vi "ps180-Rnn.vi"(3 "error in (no error)":errorcluster, 4 "Polarity":bool, 5 "Read parameter":u16 max=21 step=1, 6 "VISA session":refnum<visa-resource-name>) -> (0 "error out":errorcluster, 1 "Output string":string)   [LabVIEW 2019]
panel:
  # "Rnn, not exactly"
  # "This Vi is a kludge, don't use this to read any parameters.\nI wrote this to clone a particular operation. The numbers \nunder \"Read parameter\" don't correspond to the Rnn command\nnumbers. - MVC"
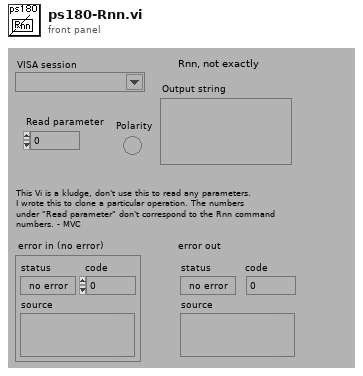
[diagram p1: front panel]
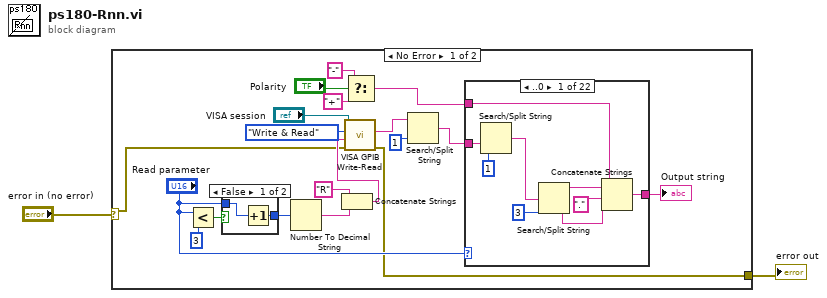
[diagram p0: block diagram]
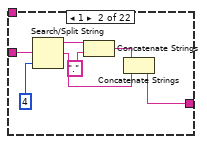
[diagram p3: hidden frame]
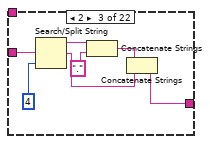
[diagram p4: hidden frame]
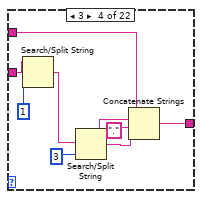
[diagram p5: hidden frame]
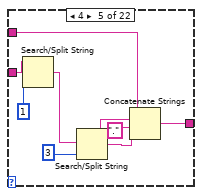
[diagram p6: hidden frame]
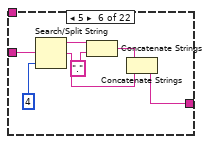
[diagram p7: hidden frame]
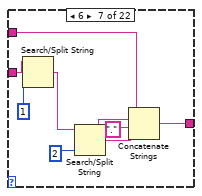
[diagram p8: hidden frame]
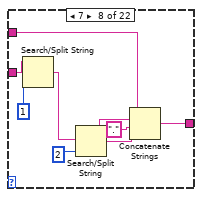
[diagram p9: hidden frame]
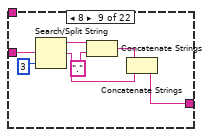
[diagram p10: hidden frame]
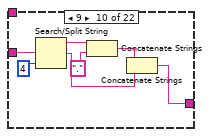
[diagram p11: hidden frame]
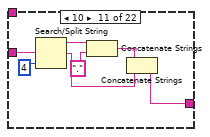
[diagram p12: hidden frame]
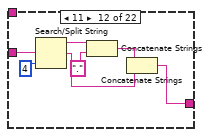
[diagram p13: hidden frame]
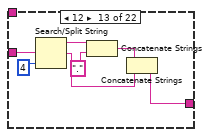
[diagram p14: hidden frame]
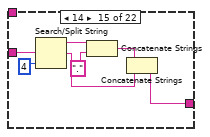
[diagram p16: hidden frame]
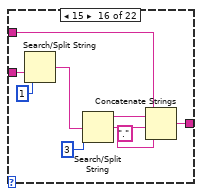
[diagram p17: hidden frame]
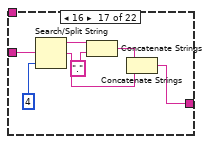
[diagram p18: hidden frame]
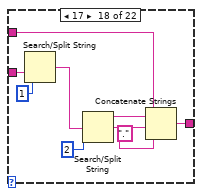
[diagram p19: hidden frame]
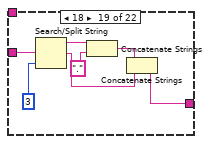
[diagram p20: hidden frame]
diagram:
  n1 = case shown="No Error" "error in (no error)" {
    selector: "error in (no error)" -> [w3 w181]
    tunnel: [w6 w181] -> w2
    frame No Error {
      n2 = Less?(x="Read parameter", y=u16 3) -> (x < y?=w10:bool)
      n3 = case shown="False" w10 {
        tunnel: "Read parameter" -> [w22 w24]
        tunnel: [w23 w24] -> w11
        frame False {
          n4 = Increment(x=w22) -> (x+1=w23:u16)
        }
        frame True {
        }
      }
      n5 = Number To Decimal String(number=w11) -> (decimal integer string=w12:string)  [unwired: 1 in]
      n6 = Concatenate Strings("R", w12) -> (w8:string)
      n7 = call "VISA GPIB Write-Read.vi"("error in (no error)"=w3, "Command"=w8, "Action"=enum16{"Write", "Read", "Write & Read"}."Write & Read", "VISA resource name"="VISA session") -> ("error out"=w6:errorcluster, "String Returned"=w7:string)  [unwired: 4 in, 2 out]
      n8 = Select(t="-", s="Polarity", f="+") -> (s? t:f=w19:string)
      n9 = Search/Split String(string=w7, offset (0)=1) -> (match + rest of string=w16:string)  [unwired: 1 in, 2 out]
      n10 = case shown="..0" "Read parameter" {
        tunnel: w16 -> [w30 w40 w42 w51 w60 w67 w76 w85 w92 w99 w106 w113 w120 w126 w128 w139 w144 w155 w160 w166 w168 w175]
        tunnel: [w28 w34 w41 w53 w62 w66 w78 w87 w91 w98 w105 w112 w119 w126 w127 w137 w143 w153 w159 w166 w167 w174] -> w17
        tunnel: w19 -> [w25 _ _ w48 w57 _ w73 w82 _ _ _ _ _ _ _ w134 _ w150 _ _ _ _]
        frame ..0 {
          n11 = Search/Split String(string=w30, offset (0)=1) -> (match + rest of string=w29:string)  [unwired: 1 in, 2 out]
          n12 = Search/Split String(string=w29, offset (0)=3) -> (substring before match=w27:string, match + rest of string=w26:string)  [unwired: 1 in, 1 out]
          n13 = Concatenate Strings(w25, w27, ".", w26) -> (w28:string)
        }
        frame 1 {
          n14 = Search/Split String(string=w40, offset (0)=4) -> (substring before match=w38:string, match + rest of string=w35:string)  [unwired: 1 in, 1 out]
          n15 = Concatenate Strings(w38, ".") -> (w36:string)
          n16 = Concatenate Strings(w36, w35) -> (w34:string)
        }
        frame 2 {
          n17 = Search/Split String(string=w42, offset (0)=4) -> (substring before match=w46:string, match + rest of string=w43:string)  [unwired: 1 in, 1 out]
          n18 = Concatenate Strings(w46, ".") -> (w44:string)
          n19 = Concatenate Strings(w44, w43) -> (w41:string)
        }
        frame 3 {
          n20 = Search/Split String(string=w51, offset (0)=1) -> (match + rest of string=w50:string)  [unwired: 1 in, 2 out]
          n21 = Search/Split String(string=w50, offset (0)=3) -> (substring before match=w55:string, match + rest of string=w52:string)  [unwired: 1 in, 1 out]
          n22 = Concatenate Strings(w48, w55, ".", w52) -> (w53:string)
        }
        frame 4 {
          n23 = Search/Split String(string=w60, offset (0)=1) -> (match + rest of string=w59:string)  [unwired: 1 in, 2 out]
          n24 = Search/Split String(string=w59, offset (0)=3) -> (substring before match=w64:string, match + rest of string=w61:string)  [unwired: 1 in, 1 out]
          n25 = Concatenate Strings(w57, w64, ".", w61) -> (w62:string)
        }
        frame 5 {
          n26 = Search/Split String(string=w67, offset (0)=4) -> (substring before match=w71:string, match + rest of string=w68:string)  [unwired: 1 in, 1 out]
          n27 = Concatenate Strings(w71, ".") -> (w69:string)
          n28 = Concatenate Strings(w69, w68) -> (w66:string)
        }
        frame 6 {
          n29 = Search/Split String(string=w76, offset (0)=1) -> (match + rest of string=w75:string)  [unwired: 1 in, 2 out]
          n30 = Search/Split String(string=w75, offset (0)=2) -> (substring before match=w80:string, match + rest of string=w77:string)  [unwired: 1 in, 1 out]
          n31 = Concatenate Strings(w73, w80, ".", w77) -> (w78:string)
        }
        frame 7 {
          n32 = Search/Split String(string=w85, offset (0)=1) -> (match + rest of string=w84:string)  [unwired: 1 in, 2 out]
          n33 = Search/Split String(string=w84, offset (0)=2) -> (substring before match=w89:string, match + rest of string=w86:string)  [unwired: 1 in, 1 out]
          n34 = Concatenate Strings(w82, w89, ".", w86) -> (w87:string)
        }
        frame 8 {
          n35 = Search/Split String(string=w92, offset (0)=3) -> (substring before match=w96:string, match + rest of string=w93:string)  [unwired: 1 in, 1 out]
          n36 = Concatenate Strings(w96, ".") -> (w94:string)
          n37 = Concatenate Strings(w94, w93) -> (w91:string)
        }
        frame 9 {
          n38 = Search/Split String(string=w99, offset (0)=4) -> (substring before match=w103:string, match + rest of string=w100:string)  [unwired: 1 in, 1 out]
          n39 = Concatenate Strings(w103, ".") -> (w101:string)
          n40 = Concatenate Strings(w101, w100) -> (w98:string)
        }
        frame 10 {
          n41 = Search/Split String(string=w106, offset (0)=4) -> (substring before match=w110:string, match + rest of string=w107:string)  [unwired: 1 in, 1 out]
          n42 = Concatenate Strings(w110, ".") -> (w108:string)
          n43 = Concatenate Strings(w108, w107) -> (w105:string)
        }
        frame 11 {
          n44 = Search/Split String(string=w113, offset (0)=4) -> (substring before match=w117:string, match + rest of string=w114:string)  [unwired: 1 in, 1 out]
          n45 = Concatenate Strings(w117, ".") -> (w115:string)
          n46 = Concatenate Strings(w115, w114) -> (w112:string)
        }
        frame 12 {
          n47 = Search/Split String(string=w120, offset (0)=4) -> (substring before match=w124:string, match + rest of string=w121:string)  [unwired: 1 in, 1 out]
          n48 = Concatenate Strings(w124, ".") -> (w122:string)
          n49 = Concatenate Strings(w122, w121) -> (w119:string)
        }
        frame 13 {
        }
        frame 14 {
          n50 = Search/Split String(string=w128, offset (0)=4) -> (substring before match=w132:string, match + rest of string=w129:string)  [unwired: 1 in, 1 out]
          n51 = Concatenate Strings(w132, ".") -> (w130:string)
          n52 = Concatenate Strings(w130, w129) -> (w127:string)
        }
        frame 15 {
          n53 = Search/Split String(string=w139, offset (0)=1) -> (match + rest of string=w138:string)  [unwired: 1 in, 2 out]
          n54 = Search/Split String(string=w138, offset (0)=3) -> (substring before match=w136:string, match + rest of string=w135:string)  [unwired: 1 in, 1 out]
          n55 = Concatenate Strings(w134, w136, ".", w135) -> (w137:string)
        }
        frame 16 {
          n56 = Search/Split String(string=w144, offset (0)=4) -> (substring before match=w148:string, match + rest of string=w145:string)  [unwired: 1 in, 1 out]
          n57 = Concatenate Strings(w148, ".") -> (w146:string)
          n58 = Concatenate Strings(w146, w145) -> (w143:string)
        }
        frame 17 {
          n59 = Search/Split String(string=w155, offset (0)=1) -> (match + rest of string=w154:string)  [unwired: 1 in, 2 out]
          n60 = Search/Split String(string=w154, offset (0)=2) -> (substring before match=w152:string, match + rest of string=w151:string)  [unwired: 1 in, 1 out]
          n61 = Concatenate Strings(w150, w152, ".", w151) -> (w153:string)
        }
        frame 18 {
          n62 = Search/Split String(string=w160, offset (0)=3) -> (substring before match=w164:string, match + rest of string=w161:string)  [unwired: 1 in, 1 out]
          n63 = Concatenate Strings(w164, ".") -> (w162:string)
          n64 = Concatenate Strings(w162, w161) -> (w159:string)
        }
        frame 19 {
        }
        frame 20 {
          n65 = Search/Split String(string=w168, offset (0)=4) -> (substring before match=w172:string, match + rest of string=w169:string)  [unwired: 1 in, 1 out]
          n66 = Concatenate Strings(w172, ".") -> (w170:string)
          n67 = Concatenate Strings(w170, w169) -> (w167:string)
        }
        frame 21.. {
          n68 = Search/Split String(string=w175, offset (0)=4) -> (substring before match=w179:string, match + rest of string=w176:string)  [unwired: 1 in, 1 out]
          n69 = Concatenate Strings(w179, ".") -> (w177:string)
          n70 = Concatenate Strings(w177, w176) -> (w174:string)
        }
      }
      "Output string" <- w17
    }
    frame Error {
    }
  }
  "error out" <- w2
